vi "svl_Log View for Resampled Energy Level (N Ch) (single value).vi"(7 "even angle channel info":T1[](array[typedef]) {"channel info"."pregain" format="%.2f"; "channel info"."weighting filter" items=["Linear", "A-weighting", "B-weighting", "C-weighting", "ITU-R 468-4", "Dolby", "CCITT", "C-message", "Wb", "Wc", "Wd", "We", "Wf", "Wh", "Wj", "Wk", "Wm", "AES17 20 kHz lowpass", "AES17 40 kHz lowpass", "AES17 20 kHz highpass", "AES17 40 kHz highpass"]; "channel info"."dB reference" format="%^.1e"; "channel info"."engineering units" items=["custom..."=0, "V"=1, "A"=21, "C"=30, "pC"=31, "s"=32, "-"=29, "Pa"=2, "N"=20, "g"=3, "m/s^2"=4, "m/s"=5, "m"=6, "mm/s"=12, "mm"=13, "micron/s"=14, "micron"=15, "in/s^2"=7, "in/s"=8, "in"=9, "mil/s"=10, "mil"=11, "rad/s^2"=16, "rad/s"=17, "rad"=18, "deg/s^2"=26, "deg/s"=27, "deg"=28, "RPM"=22, "cycle/s^2"=23, "Hz"=24, "cycle"=25, "strain"=19]; "channel info"."sensor sensitivity" format="%#_5f"}, 8 "error in (no error)":errorcluster, 9 "view mode":enum16{"Power", "Amplitude"}(ring), 10 "dB On (T)":bool=TRUE, 11 "energy levels [EU^2 rms]":dbl[](array[numeric]) format="%.2f") -> (0 "error out":errorcluster, 2 "unit label [ ]":string[](array[string]), 3 "energy levels [EU^2 rms]":dbl[](array[numeric]) format="%.2f")   [LabVIEW 2017]
uses:
  <vilib>/addons/_NISVFA/_Shared subVIs/Controls/svc_Resampled Channel Info.ctl
  <vilib>/addons/_NISVFA/_Shared subVIs/Controls/svc_Channel Info.ctl
  <vilib>/addons/_NISVFA/_Shared subVIs/Controls/svc_Engineering Units Text Ring.ctl
  <vilib>/addons/_NISVFA/_Shared subVIs/Controls/svc_Weighting Filter Text Ring.ctl
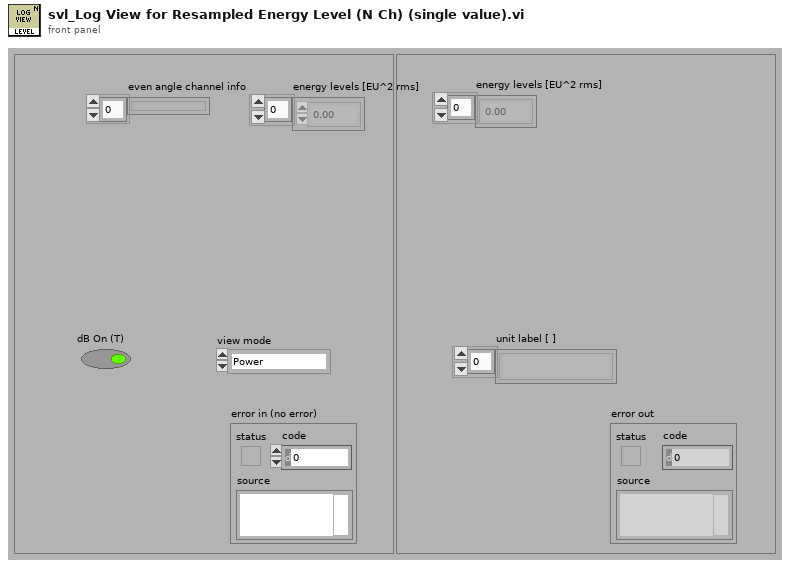
[diagram p1: front panel]
types:
  T1 = typedef "svc_Resampled Channel Info.ctl" = cluster{"channel name":string, "description":string, " channel info":T2}
  T2 = typedef "svc_Channel Info.ctl" = cluster{"sensor sensitivity":dbl, "engineering units":T3, "dB reference":dbl, "custom label":string, "weighting filter":T4, "pregain":dbl}
  T3 = typedef "svc_Engineering Units Text Ring.ctl" = u16
  T4 = typedef "svc_Weighting Filter Text Ring.ctl" = u16
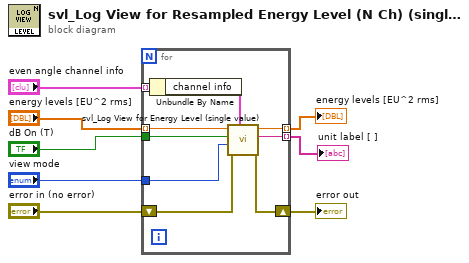
[diagram p0: block diagram]
diagram:
  n1 = for {
    tunnel: "energy levels [EU^2 rms]" -> [w16] mode=indexing
    tunnel: "dB On (T)" -> [w14]
    tunnel: "even angle channel info" -> [w11] mode=indexing
    tunnel: [w15] -> w6 mode=indexing
    tunnel: [w13] -> w5 mode=indexing
    shift-right: [w17] -> w2
    shift-left: "error in (no error)" -> [w9]
    tunnel: "view mode" -> [w12]
    n2 = Unbundle By Name(w11) -> ("channel info"=w10:T2)
    n3 = call <vilib>:"svl_Log View for Energy Level (single value).vi"("channel info"=w10, "error in (no error)"=w9, "view mode"=w12, "dB On (T)"=w14, "energy level [EU^2 rms]"=w16) -> ("error out"=w17:errorcluster, "unit label"=w13:string, "energy level [EU^2 rms]"=w15:dbl)  [unwired: 4 in]
  }
  "unit label [ ]" <- w5
  "energy levels [EU^2 rms]" <- w6
  "error out" <- w2
